vi "GetDateTime.vi"() -> (0 "date&time":string)   [LabVIEW 2015]
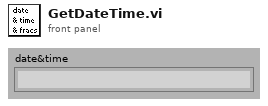
[diagram p1: front panel]
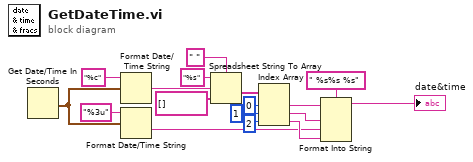
[diagram p0: block diagram]
diagram:
  n1 = Get Date/Time In Seconds() -> (seconds since 1Jan1904=w3:timestamp)
  n2 = Format Date/Time String(time format string (%c)="%c", seconds (now)=w3) -> (date/time string=w4:string)  [unwired: 1 in]
  n3 = Format Date/Time String(time format string (%c)="%3u", seconds (now)=w3) -> (date/time string=w14:string)  [unwired: 1 in]
  n4 = Spreadsheet String To Array(delimiter (Tab)=" ", format string="%s", spreadsheet string=w4, array type (2D Dbl)=string[] []) -> (array=w8:string[])
  n5 = Index Array(array=w8, index #1=0 ("index"), index #2=1 ("index"), index #3=2 ("index")) -> (element #1=w12:string, element #2=w13:string, element #3=w15:string)
  n6 = Format Into String(format string=" %s%s %s", initial string=w12, w13, w14, w15) -> (resulting string=→"date&time":string)  [unwired: 1 in, 1 out]
